vi "wherestheline.vi"(0 "SCin":u16=15000 min=10240 max=19650 step=100, 1 "S1in":u16=15000 min=10240 max=19650 step=100, 2 "S2in":u16=15000 min=10240 max=19650 step=100, 3 "S3in":u16=15000 min=10240 max=19650 step=100, 4 "S4in":u16=15000 min=10240 max=19650 step=100, 5 "S5in":u16=15000 min=10240 max=19650 step=100, 7 "last error":dbl=15000.0 min=10240.0 max=19650.0 step=100.0) -> (19 "SC":bool, 20 "error":dbl, 21 "line found":bool, 22 "really lost":bool, 23 "S1":bool, 24 "S2":bool, 25 "S3":bool, 26 "S4":bool, 27 "S5":bool)   [LabVIEW 2011]
panel:
  out "orS4":bool
  out "orS2":bool
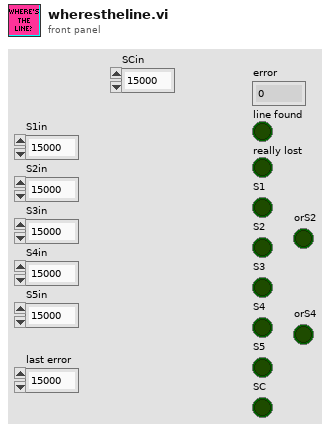
[diagram p1: front panel]
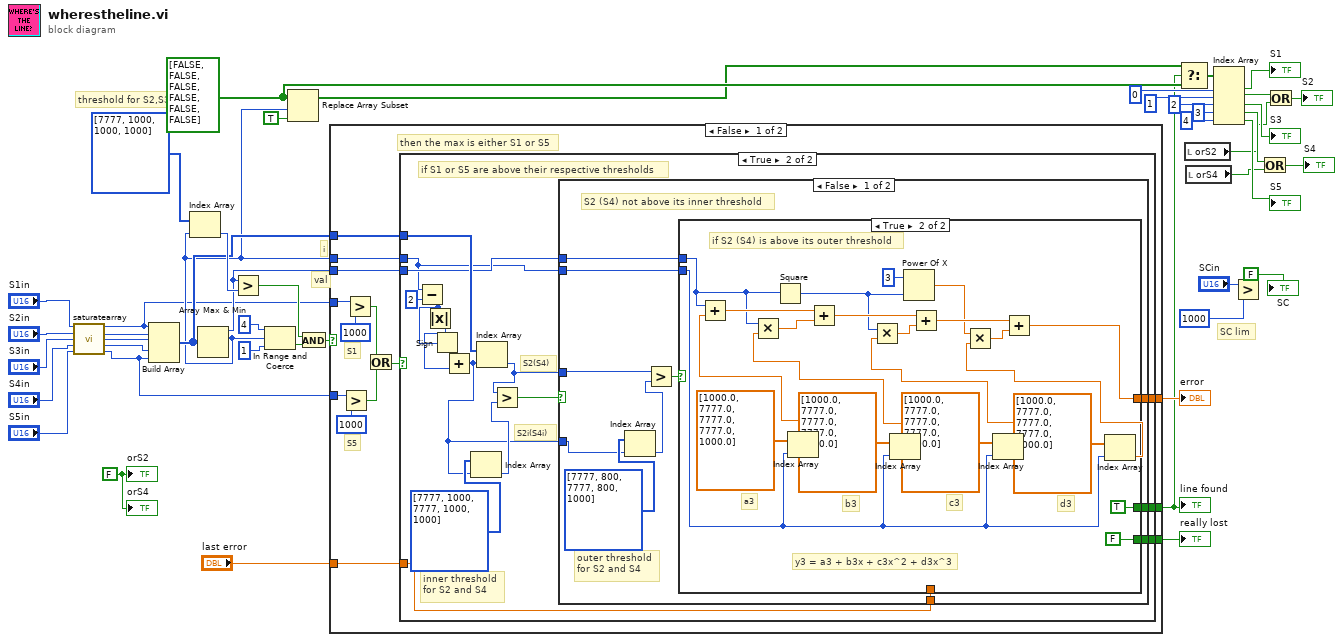
[diagram p0: block diagram]
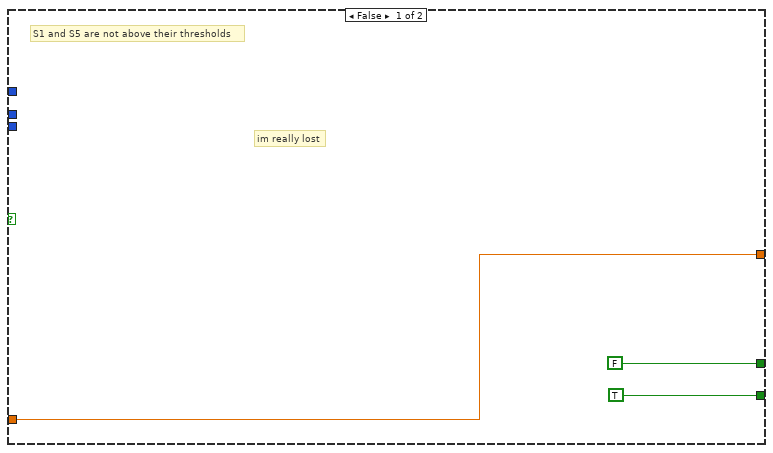
[diagram p2: hidden frame]
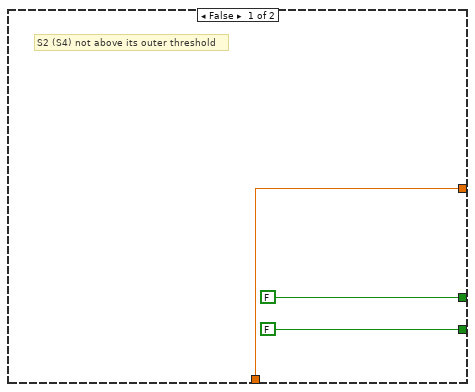
[diagram p3: hidden frame]
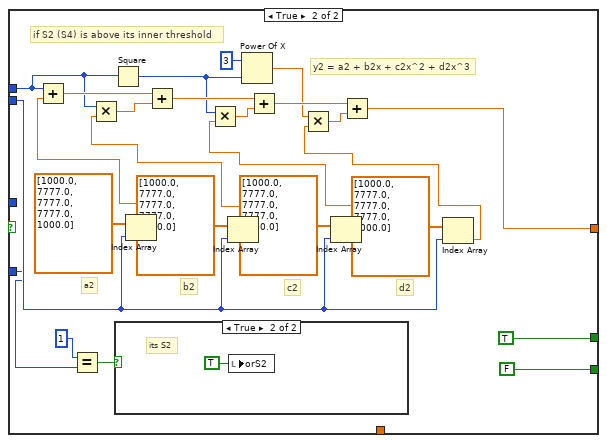
[diagram p4: hidden frame]
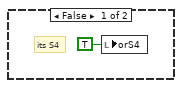
[diagram p5: hidden frame]
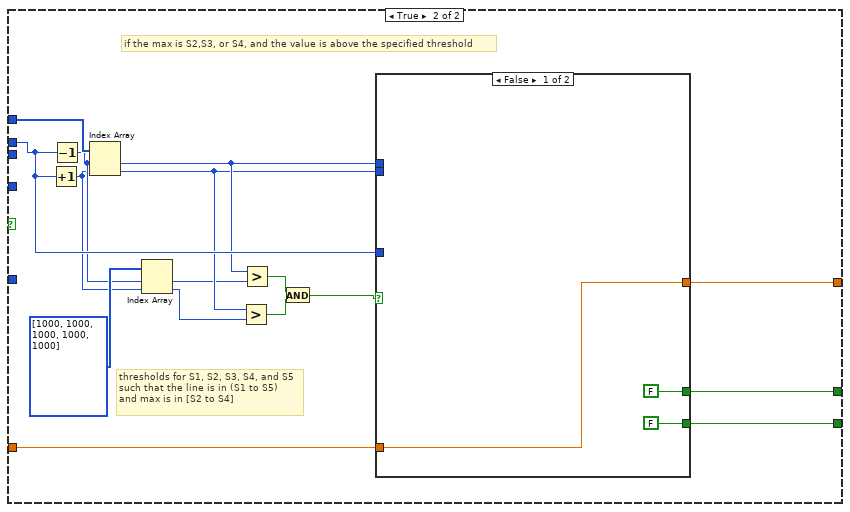
[diagram p6: hidden frame]
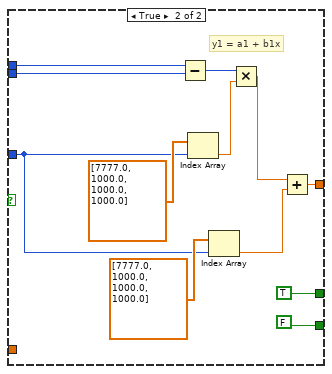
[diagram p7: hidden frame]
diagram:
  w22 = FALSE ("orS2")
  w32 = bool[] [FALSE, FALSE, FALSE, FALSE, FALSE, FALSE]
  # "SC lim"
  # "val"
  # "i"
  # "threshold for S2,S3,S4"
  n1 = call "saturatearray.vi"("S1in in"="S1in", "S2in in"="S2in", "S3in in"="S3in", "S4in in"="S4in", "S5in in"="S5in") -> ("S1in out"=w11:u16, "S2in out"=w10:u16, "S3in out"=w9:u16, "S4in out"=w8:u16, "S5in out"=w2:u16)  [unwired: 6 in]
  n2 = Build Array(w11, w10, w9, w8, w2) -> (w39:u16[])
  n3 = Array Max & Min(array=w39) -> (max value=w35:u16, max index (indices)=w34:i32)  [unwired: 2 out]
  n4 = Index Array(array=i32[] [7777, 1000, 1000, 1000], index=w34) -> (element=w41:i32)
  n5 = Greater?(x=w35, y=w41) -> (0:w42:bool)
  n6 = In Range and Coerce(upper limit=4, x=w34, lower limit=1) -> (In Range?=w43:bool)  [unwired: 1 out]
  n7 = Replace Array Subset(array=w32, new element=TRUE ("new element/subarray"), index=w34) -> (w23:bool[])
  n8 = And(x=w42, y=w43) -> (x .and. y?=w40:bool)
  n9 = case shown="False" w40 {
    tunnel: w34 -> [w54 w154]
    tunnel: w39 -> [w53 w155]
    tunnel: w11 -> [w57 _]
    tunnel: w35 -> [w52 _]
    tunnel: [w51 w158] -> w37
    tunnel: [w49 w156] -> w16
    tunnel: "last error" -> [w50 w143]
    tunnel: [w48 w157] -> w36
    tunnel: w2 -> [w47 _]
    frame False {
      # "S1"
      # "S5"
      # "then the max is either S1 or S5"
      n10 = Greater?(x=w47, y=u16 1000) -> (0:w55:bool)
      n11 = Greater?(x=w57, y=u16 1000) -> (0:w56:bool)
      n12 = Or(x=w56, y=w55) -> (x .or. y?=w60:bool)
      n13 = case shown="True" w60 {
        tunnel: w54 -> [_ w66]
        tunnel: w53 -> [_ w72]
        tunnel: w52 -> [_ w67]
        tunnel: [w63 w71] -> w51
        tunnel: w50 -> [w63 w69]
        tunnel: [FALSE w70] -> w49
        tunnel: [TRUE w68] -> w48
        frame False {
          # "im really lost"
          # "S1 and S5 are not above their thresholds"
        }
        frame True {
          # "S2(S4)"
          # "S2i(S4i)"
          # "inner threshold\nfor S2 and S4"
          # "if S1 or S5 are above their respective thresholds"
          n14 = Subtract(x=w66, y=2) -> (x-y=w65:i32)
          n15 = Absolute Value(x=w65) -> (abs(x)=w64:i32)
          n16 = Sign(1:w65) -> (0:w78:i32)
          n17 = Add(x=w78, y=w64) -> (x+y=w73:i32)
          n18 = Index Array(array=i32[] [7777, 1000, 7777, 1000, 1000], index=w73) -> (element=w76:i32)
          n19 = Index Array(array=w72, index=w73) -> (element=w74:u16)
          n20 = Greater?(x=w74, y=w76) -> (0:w75:bool)
          n21 = case shown="False" w75 {
            tunnel: w74 -> [w89 _]
            tunnel: w73 -> [w88 w117]
            tunnel: w67 -> [w85 w133]
            tunnel: w66 -> [w84 w128]
            tunnel: [w83 w121] -> w71
            tunnel: [w82 TRUE] -> w70
            tunnel: w69 -> [w81 _]
            tunnel: [w80 FALSE] -> w68
            frame False {
              # "S2 (S4) not above its inner threshold"
              # "outer threshold\nfor S2 and S4"
              n22 = Index Array(array=i32[] [7777, 800, 7777, 800, 1000], index=w88) -> (element=w87:i32)
              n23 = Greater?(x=w89, y=w87) -> (0:w86:bool)
              n24 = case shown="True" w86 {
                tunnel: w85 -> [_ w97]
                tunnel: w84 -> [_ w98]
                tunnel: [w92 w96] -> w83
                tunnel: [FALSE TRUE] -> w82
                tunnel: w81 -> [w92 _]
                tunnel: [FALSE FALSE] -> w80
                frame False {
                  # "S2 (S4) not above its outer threshold"
                }
                frame True {
                  # "d3"
                  # "c3"
                  # "b3"
                  # "a3"
                  # "y3 = a3 + b3x + c3x^2 + d3x^3"
                  # "if S2 (S4) is above its outer threshold"
                  n25 = Square(x=w97) -> (x^2=w102:u16)
                  n26 = Index Array(array=dbl[] [1000.0, 7777.0, 7777.0, 7777.0, 1000.0], index=w98) -> (element=w112:dbl)
                  n27 = Add(x=w97, y=w112) -> (x+y=w109:dbl)
                  n28 = Index Array(array=dbl[] [1000.0, 7777.0, 7777.0, 7777.0, 1000.0], index=w98) -> (element=w110:dbl)
                  n29 = Multiply(x=w97, y=w110) -> (x*y=w111:dbl)
                  n30 = Add(x=w109, y=w111) -> (x+y=w107:dbl)
                  n31 = Power Of X(1:w102, 2:3 ("y")) -> (0:w100:dbl)
                  n32 = Index Array(array=dbl[] [1000.0, 7777.0, 7777.0, 7777.0, 1000.0], index=w98) -> (element=w108:dbl)
                  n33 = Multiply(x=w102, y=w108) -> (x*y=w106:dbl)
                  n34 = Add(x=w107, y=w106) -> (x+y=w103:dbl)
                  n35 = Index Array(array=dbl[] [1000.0, 7777.0, 7777.0, 7777.0, 1000.0], index=w98) -> (element=w99:dbl)
                  n36 = Multiply(x=w100, y=w99) -> (x*y=w104:dbl)
                  n37 = Add(x=w103, y=w104) -> (x+y=w96:dbl)
                }
              }
            }
            frame True {
              # "d2"
              # "c2"
              # "b2"
              # "a2"
              # "y2 = a2 + b2x + c2x^2 + d2x^3"
              # "if S2 (S4) is above its inner threshold"
              n38 = Equal?(x=u16 1 ("t"), y=w117) -> (x = y?=w116:bool)
              n39 = Square(x=w133) -> (x^2=w125:u16)
              n40 = case shown="True" w116 {
                frame False {
                  # "its S4"
                  n41 = local write "orS4"(TRUE ("orS2")) -> ()
                }
                frame True {
                  # "its S2"
                  n42 = local write "orS2"(TRUE ("orS2")) -> ()
                }
              }
              n43 = Index Array(array=dbl[] [1000.0, 7777.0, 7777.0, 7777.0, 1000.0], index=w128) -> (element=w137:dbl)
              n44 = Add(x=w133, y=w137) -> (x+y=w134:dbl)
              n45 = Index Array(array=dbl[] [1000.0, 7777.0, 7777.0, 7777.0, 1000.0], index=w128) -> (element=w135:dbl)
              n46 = Multiply(x=w133, y=w135) -> (x*y=w136:dbl)
              n47 = Add(x=w134, y=w136) -> (x+y=w131:dbl)
              n48 = Power Of X(1:w125, 2:3 ("y")) -> (0:w123:dbl)
              n49 = Index Array(array=dbl[] [1000.0, 7777.0, 7777.0, 7777.0, 1000.0], index=w128) -> (element=w132:dbl)
              n50 = Multiply(x=w125, y=w132) -> (x*y=w130:dbl)
              n51 = Add(x=w131, y=w130) -> (x+y=w126:dbl)
              n52 = Index Array(array=dbl[] [1000.0, 7777.0, 7777.0, 7777.0, 1000.0], index=w128) -> (element=w122:dbl)
              n53 = Multiply(x=w123, y=w122) -> (x*y=w127:dbl)
              n54 = Add(x=w126, y=w127) -> (x+y=w121:dbl)
            }
          }
        }
      }
    }
    frame True {
      # "thresholds for S1, S2, S3, S4, and S5\nsuch that the line is in (S1 to S5)\nand max is in [S2 to S4]"
      # "if the max is S2,S3, or S4, and the value is above the specified threshold"
      n55 = Increment(x=w154) -> (x+1=w150:i32)
      n56 = Decrement(x=w154) -> (x-1=w151:i32)
      n57 = Index Array(array=w155, index #1=w151, index #2=w150) -> (element #1=w153:u16, element #2=w149:u16)
      n58 = Index Array(array=i32[] [1000, 1000, 1000, 1000, 1000], index #1=w151, index #2=w150) -> (element #1=w148:i32, element #2=w147:i32)
      n59 = Greater?(x=w149, y=w147) -> (0:w145:bool)
      n60 = Greater?(x=w153, y=w148) -> (0:w146:bool)
      n61 = And(x=w146, y=w145) -> (x .and. y?=w144:bool)
      n62 = case shown="False" w144 {
        tunnel: [w159 w168] -> w158
        tunnel: [FALSE ("new element/subarray") FALSE] -> w157
        tunnel: [FALSE ("new element/subarray") TRUE] -> w156
        tunnel: w153 -> [_ w164]
        tunnel: w149 -> [_ w163]
        tunnel: w154 -> [_ w162]
        tunnel: w143 -> [w159 _]
        frame False {
        }
        frame True {
          # "y1 = a1 + b1x"
          # "b1"
          # "a1"
          n63 = Subtract(x=w164, y=w163) -> (x-y=w165:u16)
          n64 = Index Array(array=dbl[] [7777.0, 1000.0, 1000.0, 1000.0], index=w162) -> (element=w171:dbl)
          n65 = Index Array(array=dbl[] [7777.0, 1000.0, 1000.0, 1000.0], index=w162) -> (element=w170:dbl)
          n66 = Multiply(x=w165, y=w171) -> (x*y=w169:dbl)
          n67 = Add(x=w169, y=w170) -> (x+y=w168:dbl)
        }
      }
    }
  }
  "error" <- w37
  "line found" <- w16
  "really lost" <- w36
  n68 = Select(t=w23, s=w16, f=w32) -> (s? t:f=w31:bool[])
  n69 = local read "orS2"() -> (w15:bool)
  n70 = local read "orS4"() -> (w14:bool)
  n71 = Index Array(array=w31, index #1=0 ("index"), index #2=1 ("index"), index #3=2 ("index"), index #4=3 ("index"), index #5=4 ("index")) -> (element #1=→"S1":bool, element #2=w18:bool, element #3=→"S3":bool, element #4=w20:bool, element #5=→"S5":bool)
  n72 = Greater?(x="SCin", y=u16 1000) -> ()  [unwired: 1 out]
  n73 = Or(x=w20, y=w14) -> (x .or. y?=→"S4":bool)
  n74 = Or(x=w18, y=w15) -> (x .or. y?=→"S2":bool)
  "SC" <- FALSE ("SC")
  "orS2" <- w22
  "orS4" <- w22
